vi "OCV Configure Acquisition.vi"(6 "Chop":bool=TRUE, 7 "Rate (Hz)":dbl=1000.0 format="%#_13g", 8 "error in (no error)":errorcluster, 9 "Min Voltage":dbl=-10.0, 10 "Max Voltage":dbl=10.0, 11 "Physical Channel":tag="4309_1/ai0:7,4309_2/ai0:7,4309_3/ai0:7") -> (0 "error out":errorcluster, 3 "Refnum out":refnum<k21>, 4 "Config Time":u32)   [LabVIEW 2019]
uses:
  <vilib>/DAQmx/create/channels.llb/DAQmx Create Channel (AI-Voltage-Basic).vi
  <vilib>/DAQmx/configure/timing.llb/DAQmx Timing (Sample Clock).vi
  <resource>/objmgr/daqmx.rc
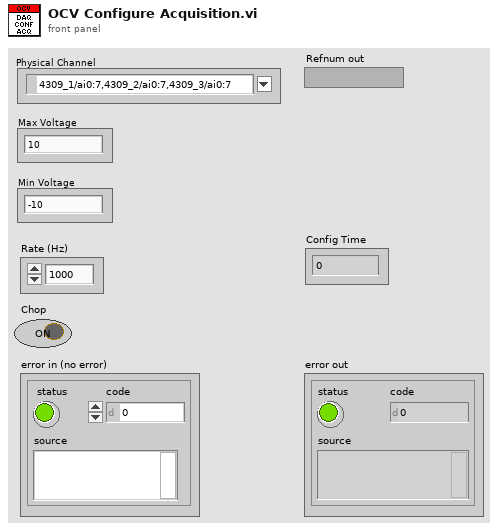
[diagram p1: front panel]
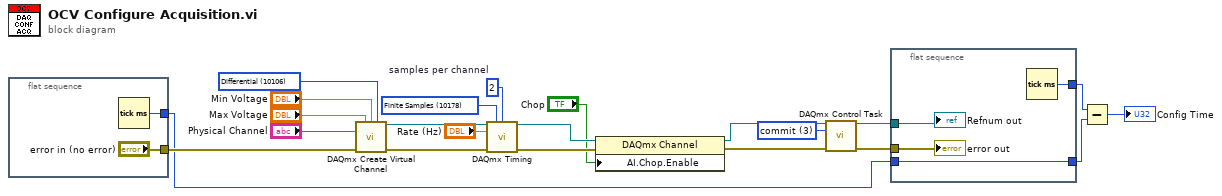
[diagram p0: block diagram]
diagram:
  w9 = 3 items=["verify"=2, "reserve"=4, "commit"=3, "unreserve"=5, "abort"=6] ("action")
  w11 = 10106 items=["default"=-1, "RSE"=10083, "NRSE"=10078, "Differential"=10106, "Pseudodifferential"=12529] ("Terminal Configuration")
  w21 = 2  # samples per channel
  w20 = 10178 items=["Finite Samples"=10178, "Continuous Samples"=10123, "Hardware Timed Single Point"=12522] ("sample mode")
  n1 = flat-sequence {
    tunnel: [w24] -> w4
    tunnel: ["error in (no error)"] -> w22
    frame #0 {
      n2 = Tick Count (ms)() -> (millisecond timer value=w24:u32)
    }
  }
  n3 = call-poly <vilib>:"DAQmx Create Virtual Channel.vi"("maximum value"="Max Voltage", "minimum value"="Min Voltage", "input terminal configuration"=w11, "physical channels"="Physical Channel", "error in"=w22) -> ("task out"=w18:refnum<k21>, "error out"=w15:errorcluster)  [unwired: 9 in]
  n4 = call-poly <vilib>:"DAQmx Timing.vi"("task/channels in"=w18, "sample mode"=w20, "samples per channel"=w21, "rate"="Rate (Hz)", "error in"=w15) -> ("task out"=w17:refnum<k21>, "error out"=w16:errorcluster)  [unwired: 9 in]
  n5 = property class="DAQmx Channel"(reference=w17, error in=w16, "AI.Chop.Enable"="Chop") -> (reference out=w7:refnum<k21>, error out=w8:errorcluster)
  n6 = call <vilib>:"DAQmx Control Task.vi"("task/channels in"=w7, "action"=w9, "error in"=w8) -> ("task out"=w6:refnum<k21>, "error out"=w5:errorcluster)  [unwired: 11 in]
  n7 = flat-sequence {
    tunnel: [w28] -> w3
    tunnel: w6 -> [w26]
    tunnel: w5 -> [w27]
    tunnel: w4 -> [w25]
    tunnel: [w25] -> w2
    frame #0 {
      n8 = Tick Count (ms)() -> (millisecond timer value=w28:u32)
      "Refnum out" <- w26
      "error out" <- w27
    }
  }
  n9 = Subtract(x=w3, y=w2) -> (x-y=→"Config Time":u32)
